vi "Time Limit Range.vi"(10 "Stop Time":cluster{"Hour":i32, "Min":i32, "Sec":i32}, 11 "Start Time":cluster{"Hour":i32, "Min":i32, "Sec":i32}) -> (3 "In Time Range":bool)   [LabVIEW 2015]
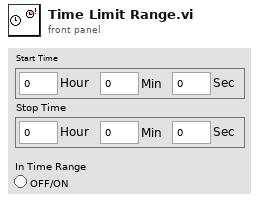
[diagram p1: front panel]
types:
  T1 = typedef "LVDateTimeRec.ctl" = cluster{"fractional second":dbl, "second":i32, "minute":i32, "hour":i32, "day of month":i32, "month":i32, "year":i32, "day of week":i32, "day of year":i32, "DST":i32}
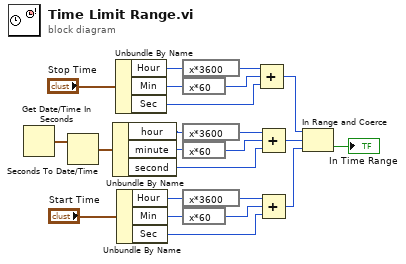
[diagram p0: block diagram]
diagram:
  n1 = Get Date/Time In Seconds() -> (seconds since 1Jan1904=w1:timestamp)
  n2 = Seconds To Date/Time(time stamp (now)=w1) -> (date time rec=w23:T1)  [unwired: 1 in]
  n3 = Unbundle By Name(w23) -> ("hour"=w20:i32, "minute"=w19:i32, "second"=w18:i32)
  n4 = Unbundle By Name("Stop Time") -> ("Hour"=w13:i32, "Min"=w12:i32, "Sec"=w11:i32)
  n5 = Unbundle By Name("Start Time") -> ("Hour"=w8:i32, "Min"=w9:i32, "Sec"=w10:i32)
  n6 = expression code="x*3600"(w13) -> (w15:i32)
  n7 = expression code="x*60"(w12) -> (w16:i32)
  n8 = expression code="x*3600"(w20) -> (w22:i32)
  n9 = expression code="x*60"(w19) -> (w21:i32)
  n10 = expression code="x*3600"(w8) -> (w7:i32)
  n11 = expression code="x*60"(w9) -> (w6:i32)
  n12 = Compound Arithmetic op=ADD(w15, w16, w11) -> (w4:i32)
  n13 = Compound Arithmetic op=ADD(w22, w21, w18) -> (w17:i32)
  n14 = Compound Arithmetic op=ADD(w7, w6, w10) -> (w3:i32)
  n15 = In Range and Coerce(upper limit=w4, x=w17, lower limit=w3) -> (In Range?=→"In Time Range":bool)  [unwired: 1 out]
